vi "Window Title.vi"(0 "LV DEV in":refnum<class "LV DEV.lvclass">, 5 "VI Reference":refnum<vi>, 11 "error in (no error)":errorcluster) -> (4 "LV DEV out":refnum<class "LV DEV.lvclass">, 6 "Window Title":string, 15 "error out":errorcluster)   [LabVIEW 2016, in "LV DEV.lvclass"]
uses:
  LV DEV.lvclass
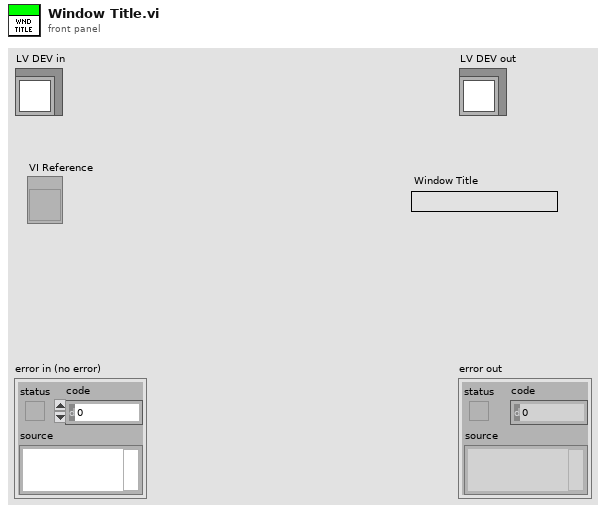
[diagram p1: front panel]
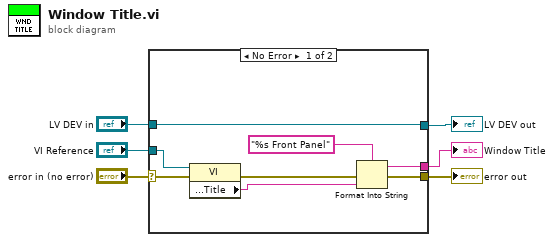
[diagram p0: block diagram]
diagram:
  n1 = case shown="No Error" "error in (no error)" {
    selector: "error in (no error)" -> [w14 w15]
    tunnel: [w9 w15] -> w5
    tunnel: [w13 w16] -> w3
    tunnel: "LV DEV in" -> [w13 w16]
    tunnel: "VI Reference" -> [w12 _]
    tunnel: [w7 _] -> w1
    frame No Error {
      n2 = property class="VI"(reference=w12, error in=w14) -> (error out=w10:errorcluster, "Front Panel.Title"=w8:string)  [unwired: 1 out]
      n3 = Format Into String(format string="%s Front Panel", error in=w10, w8) -> (resulting string=w7:string, error out=w9:errorcluster)  [unwired: 1 in]
    }
    frame Error {
    }
  }
  "error out" <- w5
  "LV DEV out" <- w3
  "Window Title" <- w1
